vi "GetIPs.vi"() -> ()   [LabVIEW 2010]
uses:
  <vilib>/Utility/file.llb/Write To Spreadsheet File (string).vi
panel:
  out "Array":string[](array[string])
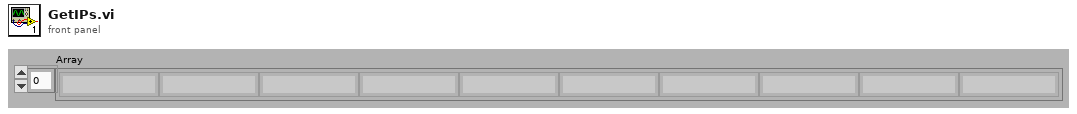
[diagram p1: front panel]
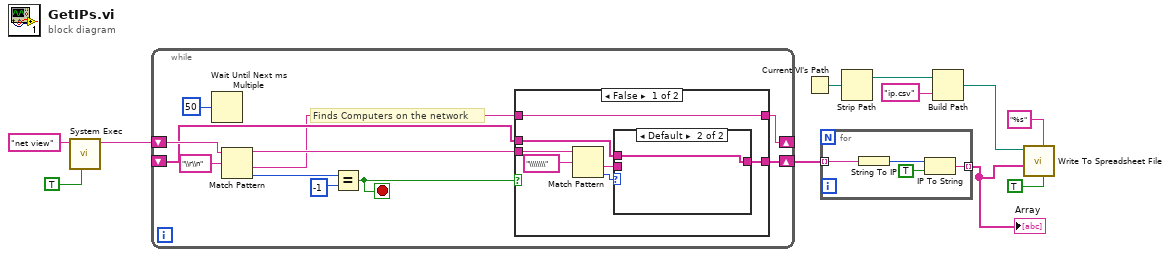
[diagram p0: block diagram]
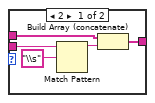
[diagram p2: hidden frame]
diagram:
  n1 = call <vilib>:"System Exec.vi"("run minimized? (F)"=TRUE, "command line"="net view") -> ("standard output"=w9:string)  [unwired: 6 in, 3 out]
  n2 = while {
    shift-right: [w13] -> _
    shift-left: w9 -> [w21]
    shift-right: [w16] -> w4
    shift-left: _ -> [w15]
    stop <- w17 stop-if-true
    # "Finds Computers on the network"
    n3 = Wait Until Next ms Multiple(millisecond multiple=u32 50) -> ()  [unwired: 1 out]
    n4 = Match Pattern(string=w21, regular expression="\\r\\n") -> (before substring=w18:string, after substring=w14:string, offset past match=w19:i32)  [unwired: 1 in, 1 out]
    n5 = Equal?(x=w19, y=-1) -> (x = y?=w17:bool)
    n6 = case shown="False" w17 {
      tunnel: w18 -> [w26 _]
      tunnel: [w25 w37] -> w16
      tunnel: w15 -> [w24 w37]
      tunnel: [w23 w36] -> w13
      tunnel: w14 -> [w23 w36]
      frame False {
        n7 = Match Pattern(string=w26, regular expression="\\\\\\\\") -> (after substring=w29:string, offset past match=w28:i32)  [unwired: 1 in, 2 out]
        n8 = case shown="Default" w28 {
          tunnel: w24 -> [w34 w35]
          tunnel: w29 -> [w32 _]
          tunnel: [w33 w35] -> w25
          frame 2 {
            n9 = Match Pattern(string=w32, regular expression="\\s") -> (before substring=w30:string)  [unwired: 1 in, 3 out]
            n10 = Build Array (concatenate)(w34, w30) -> (w33:string[])
          }
          frame Default {
          }
        }
      }
      frame True {
      }
    }
  }
  n11 = Current VI's Path() -> (path=w8:path)
  n12 = for {
    tunnel: w4 -> [w41] mode=indexing
    tunnel: [w38] -> w2 mode=indexing
    n13 = String To IP(1:w41) -> (0:w40:u32)
    n14 = IP To String(1:TRUE ("dot notation? (F)"), 2:w40) -> (0:w38:string)
  }
  "Array" <- w2
  n15 = Strip Path(path=w8) -> (stripped path=w7:path)  [unwired: 1 out]
  n16 = Build Path(base path=w7, name or relative path="ip.csv") -> (appended path=w5:path)
  n17 = call-poly <vilib>:"Write To Spreadsheet File.vi"("transpose? (no:F)"=TRUE, "format (%s)"="%s", "1D data"=w2, "file path (dialog if empty)"=w5) -> ()  [unwired: 4 in, 1 out]
